vi "main.vi"() -> ()   [LabVIEW 2025]
uses:
  1cbc7890-2b9e-4b6b-a63a-61c39f236014.vi
  9dd541fc-abbd-4630-bc63-6a61ac9cb119.vi
panel:
  out "error out 2":errorcluster
  out "fast":bool
  out "score.p2":i32
  out "score.p1":i32
  in  "Cluster":cluster{"score":cluster{"p1":i32, "p2":i32}}
  out "output cluster":cluster{i32, i32, i32}
  out "error out":errorcluster
  in  "Array":bool[](array[boolean])=[FALSE, FALSE, FALSE, FALSE, FALSE, FALSE, FALSE, FALSE, FALSE, FALSE, FALSE, FALSE, FALSE, FALSE, FALSE, FALSE, FALSE, FALSE, FALSE, FALSE, FALSE, FALSE, FALSE, FALSE, FALSE, FALSE, FALSE, FALSE, FALSE, FALSE, FALSE, FALSE, FALSE, FALSE, FALSE, FALSE, FALSE, FALSE, FALSE, FALSE, FALSE, FALSE, FALSE, FALSE, FALSE, FALSE, FALSE, FALSE, FALSE, FALSE, FALSE, FALSE, FALSE, FALSE, FALSE, FALSE, FALSE, FALSE, FALSE, FALSE, FALSE, FALSE, FALSE, FALSE, FALSE, FALSE, FALSE, FALSE, FALSE, FALSE, FALSE, FALSE, FALSE, FALSE, FALSE, FALSE, FALSE, FALSE, FALSE, FALSE, FALSE, FALSE, FALSE, FALSE, FALSE, FALSE, FALSE, FALSE, FALSE, FALSE, FALSE, FALSE, FALSE, FALSE, FALSE, FALSE, FALSE, FALSE, FALSE, FALSE]
  out "actions":string
  out "keys":bool[](array[boolean])
  in  "enter":bool
  in  "mode":u16(ring) items=["1 player", "AI vs. AI", "2 players (online)", "2 players (offline)"]
  in  "Reset":bool
  in  "Stop":bool
  out "screen":picture
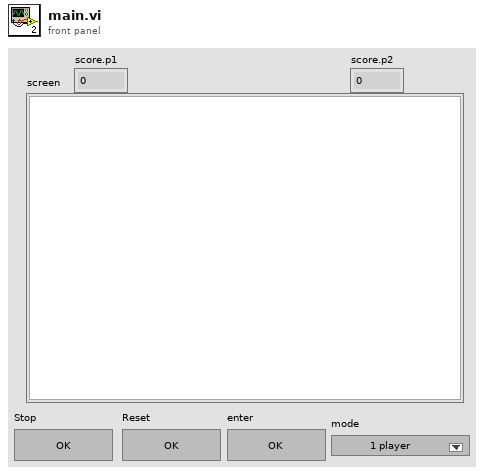
[diagram p1: front panel]
types:
  T1 = typedef "Sound Output Task ID.ctl" = u32
  T2 = cluster{"player1":cluster{"x":i32, "y":i32, "dive_direction":i32, "state":i32, "frame_num":i32}, "player2":cluster{"x":i32, "y":i32, "state":i32, "frame_num":i32, "dive_direction":i32}, "ball":cluster{"x":i32, "y":i32, "rotation":i32}, "ball_hyper":cluster{"x":i32, "y":i32, "visible":bool}, "ball_trail":cluster{"x":i32, "y":i32, "visible":bool}, "punch":cluster{"x":i32, "y":i32, "visible":bool}}
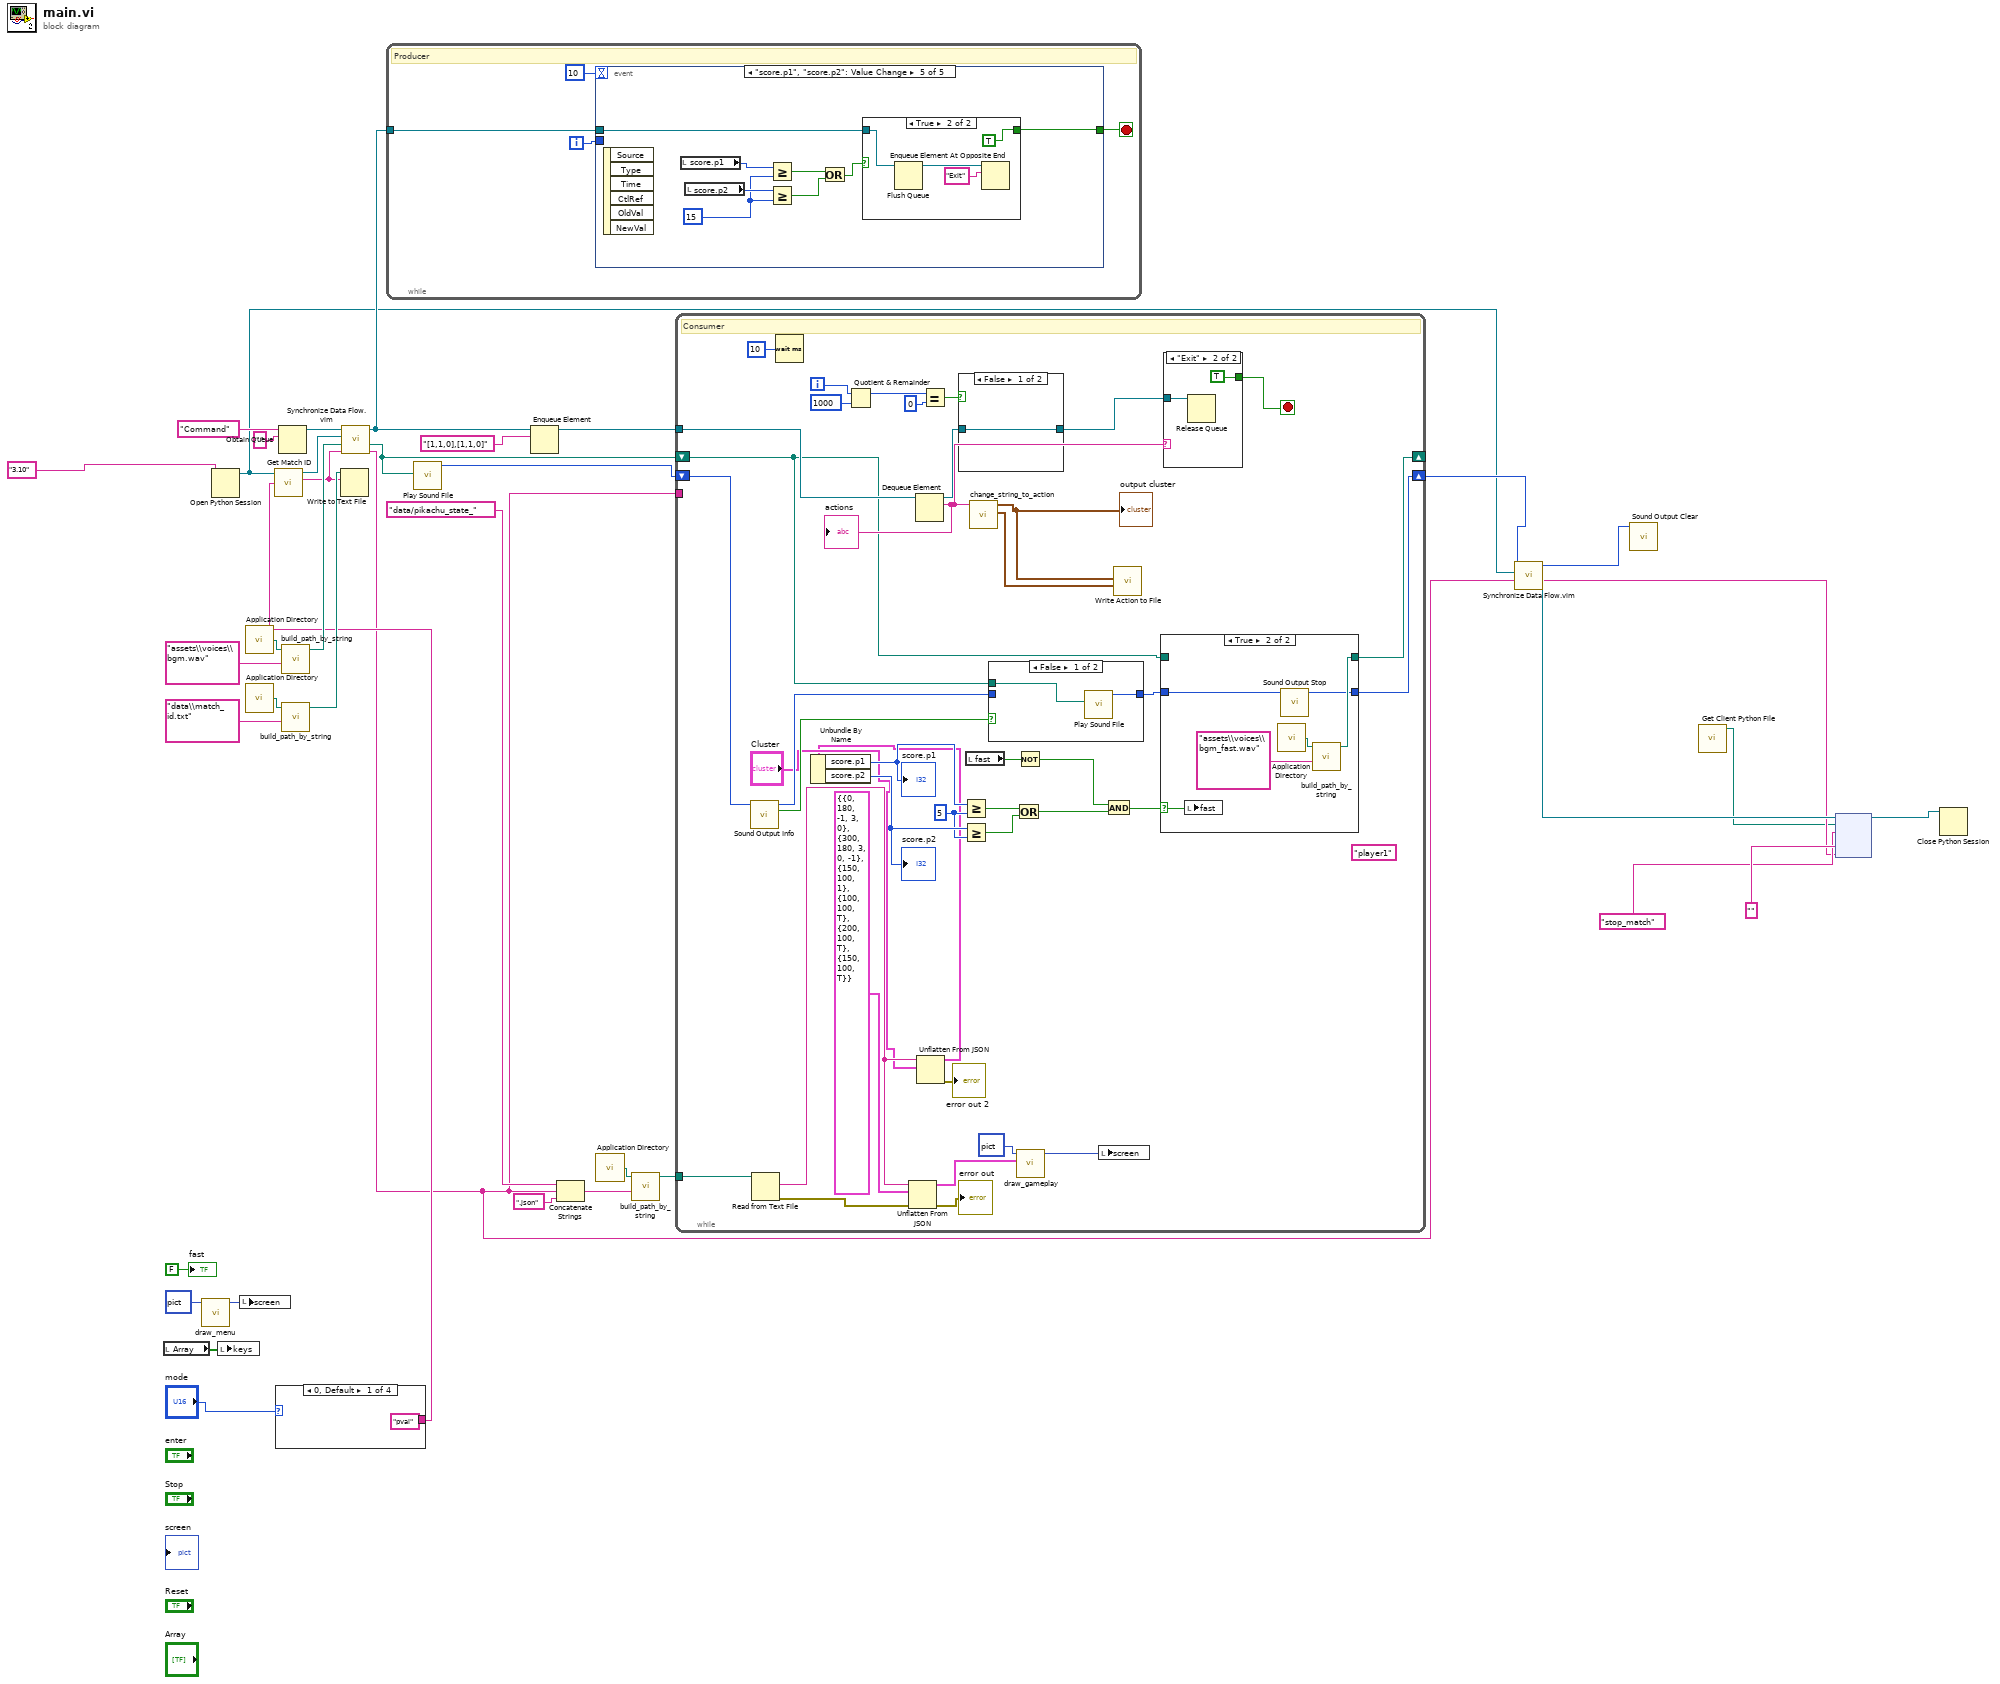
[diagram p0: block diagram]
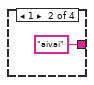
[diagram p2: hidden frame]
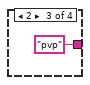
[diagram p3: hidden frame]
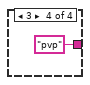
[diagram p4: hidden frame]
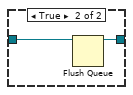
[diagram p6: hidden frame]
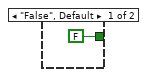
[diagram p8: hidden frame]
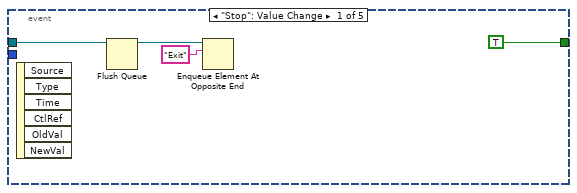
[diagram p9: hidden frame]
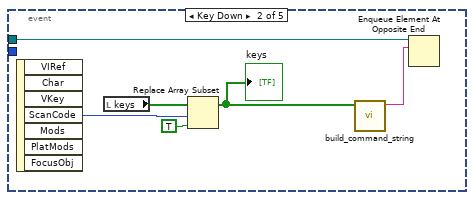
[diagram p10: hidden frame]
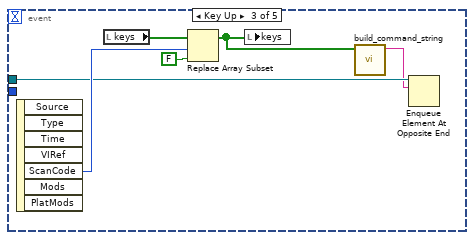
[diagram p11: hidden frame]
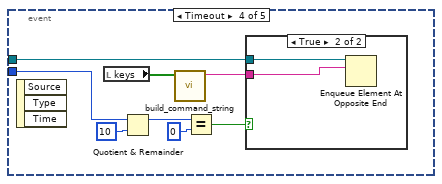
[diagram p12: hidden frame]
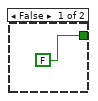
[diagram p14: hidden frame]
diagram:
  n1 = local read "Array"() -> (w38:bool[])
  n2 = call "draw_menu.vi"("input"=picture data[5B]) -> ("menu"=w37:picture)  [unwired: 10 in]
  n3 = Open Python Session(python version="3.10" ("Python version")) -> (session out=w5:refnum<k35>)  [unwired: 2 in, 1 out]
  n4 = local write "keys"(w38) -> ()
  n5 = local write "screen"(w37) -> ()
  n6 = call <vilib>:"Application Directory.vi"() -> ("Application Directory"=w35:path)
  n7 = call <vilib>:"Application Directory.vi"() -> ("Application Directory"=w27:path)
  n8 = case shown="0, Default" "mode" {
    tunnel: ["pvai" "aivai" "pvp" "pvp"] -> w12
    frame 0, Default {
    }
    frame 1 {
    }
    frame 2 {
    }
    frame 3 {
    }
  }
  n9 = call "Get Match ID.vi"("Refnum in"=w5, "mode"=w12) -> ("Refnum out"=w19:refnum<k35>, "return value"=w25:string)  [unwired: 5 in, 2 out]
  n10 = Obtain Queue(name (unnamed)="Command", element data type="" ("name (unnamed)")) -> (queue out=w33:refnum<queue>)  [unwired: 3 in, 2 out]
  n11 = call "build_path_by_string.vi"("String"="assets\\voices\\bgm.wav", "base path"=w35) -> ("appended path"=w32:path)  [unwired: 9 in]
  n12 = call "build_path_by_string.vi"("String"="data\\match_id.txt", "base path"=w27) -> ("appended path"=w26:path)  [unwired: 9 in]
  n13 = Write to Text File(file (use dialog)=w26, text=w25) -> ()  [unwired: 2 in, 3 out]
  n14 = call "Synchronize Data Flow.vim"("input 4"=w25, "input 3"=w32, "input 2"=w19, "input 1"=w33) -> ("output 4"=w6:string, "output 3"=w14:path, "output 1"=w17:refnum<queue>)  [unwired: 1 out]
  n15 = while {
    tunnel: w17 -> [w45]
    i -> [w44]
    stop <- w46 stop-if-true
    # "Producer"
    n16 = event shown="[4] \"score.p1\", \"score.p2\": Value Change" {
      selector: _ -> [_ _ _ _ _]
      dyn-events: _ -> [_ _ _ _ _]
      timeout: 10 -> [_ _ _ _ _]
      tunnel: [TRUE _ _ _ w73] -> w46
      tunnel: w45 -> [w49 w52 w58 w70 w74]
      tunnel: w44 -> [_ _ _ w67 _]
      event "Stop": Value Change {
        n17 = event-data() -> ()  [unwired: 1 in, 6 out]
        n18 = Flush Queue(queue=w49) -> (queue out=w48:refnum<queue>)  [unwired: 1 in, 2 out]
        n19 = Enqueue Element At Opposite End(queue=w48, element="Exit") -> ()  [unwired: 2 in, 3 out]
      }
      event Key Down {
        n20 = event-data() -> ("ScanCode"=w55:i16)  [unwired: 1 in, 6 out]
        n21 = local read "keys"() -> (w56:bool[])
        n22 = Replace Array Subset(array=w56, new element=TRUE ("new element/subarray"), index=w55) -> (w53:bool[])
        "keys" <- w53
        n23 = call "build_command_string.vi"("key state"=w53) -> ("command"=w51:string)  [unwired: 10 in]
        n24 = Enqueue Element At Opposite End(queue=w52, element=w51) -> ()  [unwired: 2 in, 3 out]
      }
      event Key Up {
        n25 = event-data() -> ("ScanCode"=w60:i16)  [unwired: 1 in, 6 out]
        n26 = local read "keys"() -> (w62:bool[])
        n27 = Replace Array Subset(array=w62, new element=FALSE ("new element/subarray"), index=w60) -> (w59:bool[])
        n28 = local write "keys"(w59) -> ()
        n29 = call "build_command_string.vi"("key state"=w59) -> ("command"=w57:string)  [unwired: 10 in]
        n30 = Enqueue Element At Opposite End(queue=w58, element=w57) -> ()  [unwired: 2 in, 3 out]
      }
      event Timeout {
        n31 = event-data() -> ()  [unwired: 1 in, 3 out]
        n32 = local read "keys"() -> (w68:bool[])
        n33 = Quotient & Remainder(x=w67, y=10) -> (x-y*floor(x/y)=w65:i32)  [unwired: 1 out]
        n34 = call "build_command_string.vi"("key state"=w68) -> ("command"=w69:string)  [unwired: 10 in]
        n35 = Equal?(x=w65, y=0) -> (x = y?=w64:bool)
        n36 = case shown="True" w64 {
          tunnel: w70 -> [_ w72]
          tunnel: w69 -> [_ w71]
          frame False {
          }
          frame True {
            n37 = Enqueue Element At Opposite End(queue=w72, element=w71) -> ()  [unwired: 2 in, 3 out]
          }
        }
      }
      event "score.p1", "score.p2": Value Change {
        w76 = 15
        n38 = event-data() -> ()  [unwired: 1 in, 6 out]
        n39 = local read "score.p1"() -> (w78:i32)
        n40 = local read "score.p2"() -> (w77:i32)
        n41 = Greater Or Equal?(x=w78, y=w76) -> (x >= y?=w80:bool)
        n42 = Greater Or Equal?(x=w77, y=w76) -> (x >= y?=w79:bool)
        n43 = Or(x=w80, y=w79) -> (x .or. y?=w75:bool)
        n44 = case shown="True" w75 {
          tunnel: w74 -> [_ w83]
          tunnel: [FALSE TRUE] -> w73
          frame False {
          }
          frame True {
            n45 = Flush Queue(queue=w83) -> (queue out=w85:refnum<queue>)  [unwired: 1 in, 2 out]
            n46 = Enqueue Element At Opposite End(queue=w85, element="Exit") -> ()  [unwired: 2 in, 3 out]
          }
        }
      }
    }
  }
  n47 = call <vilib>:"Play Sound File.vi"("path"=w14) -> ("task ID"=w34:T1)  [unwired: 9 in, 1 out]
  n48 = Enqueue Element(queue=w17, element="[1,1,0],[1,1,0]") -> (queue out=w16:refnum<queue>)  [unwired: 2 in, 2 out]
  n49 = Concatenate Strings("data/pikachu_state_" ("string"), w6, ".json" ("string")) -> (w21:string)
  n50 = call <vilib>:"Application Directory.vi"() -> ("Application Directory"=w22:path)
  n51 = call "build_path_by_string.vi"("String"=w21, "base path"=w22) -> ("appended path"=w20:path)  [unwired: 9 in]
  n52 = while {
    tunnel: w16 -> [w125]
    shift-right: [w92] -> w8
    shift-left: w34 -> [w120]
    tunnel: w20 -> [w117]
    tunnel: w6 -> [_]
    shift-right: [w95] -> _
    shift-left: w14 -> [w94]
    i -> [w107]
    stop <- w123 stop-if-true
    w99 = 5 ("y")
    (unwired) "player1" ("role")
    # "Consumer"
    n53 = call <vilib>:"Sound Output Info.vi"("task ID"=w120) -> ("is playing?"=w122:bool, "task ID out"=w121:T1)  [unwired: 7 in, 2 out]
    n54 = Read from Text File(file (use dialog)=w117) -> (text=w90:string, error out=w113:errorcluster)  [unwired: 3 in, 2 out]
    n55 = Wait (ms)(milliseconds to wait=u32 10) -> ()  [unwired: 1 out]
    n56 = Quotient & Remainder(x=w107, y=1000) -> (x-y*floor(x/y)=w109:i32)  [unwired: 1 out]
    n57 = Unflatten From JSON(JSON string=w90, type and defaults=T2 {"player1"={"x"=0, "y"=180, "dive_direction"=-1, "state"=3, "frame_num"=0}, "player2"={"x"=300, "y"=180, "state"=3, "frame_num"=0, "dive_direction"=-1}, "ball"={"x"=150, "y"=100, "rotation"=1}, "ball_hyper"={"x"=100, "y"=100, "visible"=TRUE}, "ball_trail"={"x"=200, "y"=100, "visible"=TRUE}, "punch"={"x"=150, "y"=100, "visible"=TRUE}} ("status"), error in (no error)=w113) -> (value=w115:T2, error out=→"error out":errorcluster)  [unwired: 4 in]
    n58 = Dequeue Element(queue=w125) -> (queue out=w112:refnum<queue>, element=w105:string)  [unwired: 2 in, 2 out]
    "actions" <- w105
    n59 = Unflatten From JSON(JSON string=w90, type and defaults="Cluster") -> (value=w88:cluster{"score":cluster{"p1":i32, "p2":i32}}, error out=→"error out 2":errorcluster)  [unwired: 5 in]
    n60 = Unbundle By Name(w88) -> ("score.p1"=w101:i32, "score.p2"=w100:i32)
    "score.p1" <- w101
    "score.p2" <- w100
    n61 = Equal?(x=w109, y=0) -> (x = y?=w106:bool)
    n62 = case shown="False" w106 {
      tunnel: w112 -> [w134 w136]
      tunnel: [w134 w135] -> w111
      frame False {
      }
      frame True {
        n63 = Flush Queue(queue=w136) -> (queue out=w135:refnum<queue>)  [unwired: 1 in, 2 out]
      }
    }
    n64 = Greater Or Equal?(x=w101, y=w99) -> (x >= y?=w98:bool)
    n65 = Greater Or Equal?(x=w100, y=w99) -> (x >= y?=w97:bool)
    n66 = local read "fast"() -> (w104:bool)
    n67 = call "change_string_to_action.vi"("String"=w105) -> ("output cluster 2"=w86:cluster{i32, i32, i32}, "output cluster"=w91:cluster{i32, i32, i32})  [unwired: 9 in]
    "output cluster" <- w91
    n68 = case shown="False" w122 {
      tunnel: w94 -> [w138 _]
      tunnel: [w137 w139] -> w93
      tunnel: w121 -> [_ w139]
      frame False {
        n69 = call <vilib>:"Play Sound File.vi"("path"=w138) -> ("task ID"=w137:T1)  [unwired: 9 in, 1 out]
      }
      frame True {
      }
    }
    n70 = Or(x=w98, y=w97) -> (x .or. y?=w96:bool)
    n71 = Not(x=w104) -> (.not. x?=w103:bool)
    n72 = call "draw_gameplay.vi"("status"=w115, "input"=picture data[5B]) -> ("gameplay"=w119:picture)  [unwired: 9 in]
    n73 = local write "screen"(w119) -> ()
    n74 = And(x=w103, y=w96) -> (x .and. y?=w102:bool)
    n75 = call "Write Action to File.vi"("action_code"=w91, "action_code 2"=w86) -> ()  [unwired: 8 in]
    n76 = case shown="True" w102 {
      selector: w102 -> [_ w133]
      tunnel: [w127 w130] -> w95
      tunnel: w94 -> [w127 _]
      tunnel: w93 -> [w126 w129]
      tunnel: [w126 w128] -> w92
      frame False {
      }
      frame True {
        n77 = local write "fast"(w133) -> ()
        n78 = call <vilib>:"Application Directory.vi"() -> ("Application Directory"=w132:path)
        n79 = call <vilib>:"Sound Output Stop.vi"("task ID"=w129) -> ("task ID out"=w128:T1)  [unwired: 9 in, 1 out]
        n80 = call "build_path_by_string.vi"("String"="assets\\voices\\bgm_fast.wav", "base path"=w132) -> ("appended path"=w130:path)  [unwired: 9 in]
      }
    }
    n81 = case shown="\"Exit\"" w105 {
      tunnel: w111 -> [_ w142]
      tunnel: [FALSE TRUE] -> w123
      frame "False", Default {
      }
      frame "Exit" {
        n82 = Release Queue(queue=w142) -> ()  [unwired: 2 in, 3 out]
      }
    }
  }
  n83 = call "Synchronize Data Flow.vim"("input 3"=w6, "input 2"=w5, "input 1"=w8) -> ("output 3"=w3:string, "output 2"=w4:refnum<k35>, "output 1"=w7:T1)  [unwired: 1 in, 1 out]
  n84 = call <vilib>:"Sound Output Clear.vi"("task ID"=w7) -> ()  [unwired: 10 in, 1 out]
  n85 = call "Get Client Python File.vi"() -> ("appended path"=w1:path)  [unwired: 11 in]
  n86 = node(w4, w1, "stop_match" ("function name"), "", w3) -> (w2:refnum<k35>)  [unwired: 3 in, 3 out]
  n87 = Close Python Session(session in=w2) -> ()  [unwired: 1 in, 1 out]
  "fast" <- FALSE ("fast")
